vi "Save Progress.vi"(11 "Internal Data In":T1) -> (3 "Internal Data Out":T1)   [LabVIEW 2025]
uses:
  Internal Data.ctl
  Collision Box.ctl
  <vilib>/picture/picture.llb/imagedata.ctl
  <vilib>/Utility/config.llb/Write Key (I32).vi
  <vilib>/Utility/config.llb/Read Key (I32).vi
  <vilib>/Utility/config.llb/NI_LVConfig.lvlib
types:
  T1 = typedef "Internal Data.ctl" = cluster{"Core":cluster{"Current VI Reference":refnum<vi>, "Close Panel on Exit?":bool}, "Collision Box":T2, "Walls":cluster{"[0]":T3, "[1]":T3, "[2]":T3, "[3]":T3, "[4]":T3, "[5]":T3, "[6]":T3, "[7]":T3, "[8]":T3}, "Floor":T3, "Gates":cluster{"[0]":T3, "[1]":T3, "[2]":T3, "[3]":T3, "[4]":T3, "[5]":T3, "[6]":T3, "[7]":T3, "[8]":T3}, "Gate Condition":bool[], "Level":i32, "Score":i32, "Player Image":T3, "Display Font":cluster{"Font Name:":string, "Size":i16, "Strikeout?":bool, "Italic?":bool, "Underline?":bool, "Outline?":bool, "Shadow?":bool, "Bold?":bool}, "Menu Image":T3, "Menu Button Image":T3, "Menu Selected Image":T3, "Menu Selection":i32, "Player Name":string, "Menu Wall Image":T3, "Up Arrow":T3, "Down Arrow":T3, "Left Arrow":T3, "Right Arrow":T3, "Record Path":path, "Toggle Audio":path, "Theme Audio":path}
  T2 = typedef "Collision Box.ctl" = cluster{"left":i16, "top":i16, "right":i16, "bottom":i16}
  T3 = typedef "imagedata.ctl" = cluster{"image type":i32, "image depth":i32, "image":u8[], "mask":u8[], "colors":u32[], "Rectangle":cluster{"left":i16, "top":i16, "right":i16, "bottom":i16}}
  T4 = typedef "NI_LVConfig.lvlib/Config Data RefNum.ctl" = refnum<k1>
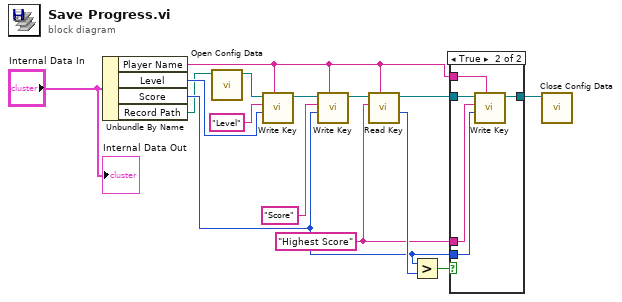
[diagram p0: block diagram]
diagram:
  w3 = "Highest Score" ("key")
  n1 = Unbundle By Name("Internal Data In") -> ("Player Name"=w4:string, "Level"=w12:i32, "Score"=w2:i32, "Record Path"=w1:path)
  n2 = call <vilib>:"Open Config Data.vi"("configuration file path"=w1) -> ("refnum"=w15:T4)  [unwired: 8 in, 2 out]
  n3 = call-poly <vilib>:"Write Key.vi"("section"=w4, "value"=w12, "key"="Level", "refnum"=w15) -> ("refnum out"=w11:T4)  [unwired: 5 in, 2 out]
  n4 = call-poly <vilib>:"Write Key.vi"("section"=w4, "value"=w2, "key"="Score", "refnum"=w11) -> ("refnum out"=w9:T4)  [unwired: 5 in, 2 out]
  n5 = call-poly <vilib>:"Read Key.vi"("section"=w4, "key"=w3, "refnum"=w9) -> ("value"=w6:i32, "refnum out"=w8:T4)  [unwired: 5 in, 2 out]
  n6 = Greater?(x=w2, y=w6) -> (0:w5:bool)
  n7 = case shown="True" w5 {
    tunnel: w8 -> [w16 w21]
    tunnel: [w16 w20] -> w7
    tunnel: w4 -> [_ w19]
    tunnel: w3 -> [_ w18]
    tunnel: w2 -> [_ w17]
    frame False {
    }
    frame True {
      n8 = call-poly <vilib>:"Write Key.vi"("section"=w19, "value"=w17, "key"=w18, "refnum"=w21) -> ("refnum out"=w20:T4)  [unwired: 5 in, 2 out]
    }
  }
  n9 = call <vilib>:"Close Config Data.vi"("refnum"=w7) -> ()  [unwired: 9 in, 2 out]
  "Internal Data Out" <- "Internal Data In"
